vi "SCI_TxPck.vi"(9 "数据有效":bool, 10 "数据类型":u16 format="%x", 11 "数据":u16 format="%x") -> (2 "CRC余数":u16 format="%x", 3 "数据包输出":T1 {"包头" format="%02x"; "数据低8位" format="%02x"; "数据低高8位" format="%02x"; "数据类型" items=["SCIDP_SPTG1"=16, "SCIDP_SPTG2"=17, "SCIDP_INSTR1"=18, "SCIDP_INSTR2"=19, "SCIDP_DTTG1"=20, "SCIDP_DTTG2"=21, "SCIDP_VRPH1"=22, "SCIDP_VRPH2"=23, "RSVD0x18"=24, "RSVD0x19"=25, "RSVD0x1A"=26, "RSVD0x1B"=27, "RSVD0x1C"=28, "RSVD0x1D"=29, "RSVD0x1E"=30, "RSVD0x1F"=31, "SCIDP_SRVST1"=32, "SCIDP_SRVST2"=33, "SCIDP_SPFB1"=34, "SCIDP_SPFB2"=35, "RSVD0x24"=36, "RSVD0x25"=37, "RSVD0x26"=38, "RSVD0x27"=39, "RSVD0x28"=40, "RSVD0x29"=41, "RSVD0x2A"=42, "RSVD0x2B"=43, "RSVD0x2C"=44, "RSVD0x2D"=45, "SCIDP_EFFC1"=46, "SCIDP_EFFC2"=47, "RSVD0x30"=48, "RSVD0x31"=49, "SCIDP_IBUS1"=50, "SCIDP_IBUS2"=51, "SCIDP_IA1"=52, "SCIDP_IA2"=53, "SCIDP_IB1"=54, "SCIDP_IB2"=55, "SCIDP_IC1"=56, "SCIDP_IC2"=57, "SCIDP_UBUS1"=58, "SCIDP_UBUS2"=59, "SCIDP_TMPR1"=60, "SCIDP_TMPR2"=61, "RSVD0x3E"=62, "RSVD0x3F"=63, "VOID"=0]; "CRC余数" format="%02x"})   [LabVIEW 2015]
uses:
  SCI_DataPck.ctl
  SCI_DataType.ctl
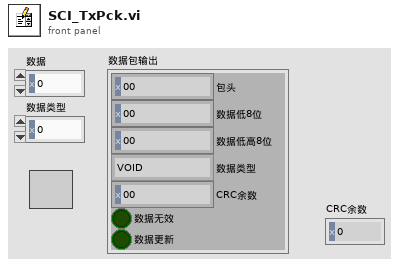
[diagram p1: front panel]
types:
  T1 = typedef "SCI_DataPck.ctl" = cluster{"包头":u16, "数据低8位":u16, "数据低高8位":u16, "数据类型":T2, "CRC余数":u16, "数据无效":bool, "数据更新":bool}
  T2 = typedef "SCI_DataType.ctl" = u16
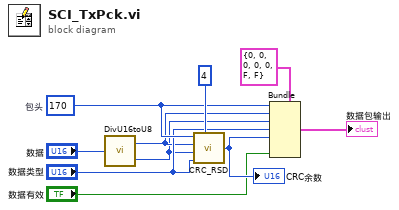
[diagram p0: block diagram]
diagram:
  w9 = u16 170  # 包头
  n1 = call "DivU16toU8.vi"("Uint16_in"="数据") -> ("Uint8L_out"=w6:u8, "Uint8H_out"=w5:u8)
  n2 = call "CRC_RSD.vi"("BYTE 0"=w9, "BYTE 1"=w6, "BYTE 2"=w5, "BYTE 3"="数据类型", "Number of BYTE"=4) -> ("RSD"=w4:u16)
  "CRC余数" <- w4
  n3 = Bundle(cluster=T1 {"包头"=0, "数据低8位"=0, "数据低高8位"=0, "数据类型"=0, "CRC余数"=0, "数据无效"=FALSE, "数据更新"=FALSE}, "包头"=w9, "数据低8位"=w6, "数据低高8位"=w5, "数据类型"="数据类型", "CRC余数"=w4, "数据更新"="数据有效") -> (→"数据包输出":T1)  [unwired: 1 in]
